vi "TEST_L1_TRANSFER_FUNCTION.vi"(5 "Serial Number":string="SN_00268", 6 "error in":errorcluster, 9 "Instrument VISA in":T1={"AWG VISA"="AgilentGen1", "Oscilloscope  VISA "="AgilentOsc", "Integration Board IP"="172.16.17.48", "connection ID"=refnum, "report out"=refnum, "report file path"=path "C:/Users/omartinez/Desktop/L0nL1_Results"}) -> (0 "error out":errorcluster, 3 "VISA Out":T1={"AWG VISA"="AgilentGen1", "Oscilloscope  VISA "="AgilentOsc", "Integration Board IP"="172.16.17.48", "connection ID"=refnum, "report out"=refnum, "report file path"=path "C:/Users/omartinez/Desktop/L0nL1_Results"})   [LabVIEW 2012]
uses:
  <vilib>/Utility/NIReport.llb/NI_report.lvclass
  <vilib>/Utility/NIReport.llb/HTML/NI_HTML.lvclass
  <instrlib>/Agilent 8000 Series/Agilent 8000 Series.lvlib
  Sum_Abrilader/L0_Sum_Adder Folder/C/Program Files/National Instruments/LabVIEW 2012/instr.lib/Agilent 81150/Agilent 81150.lvlib
panel:
  in  "SmartScan/\nLinearScan?":bool
  in  "Threshold Limits":i16[](array[numeric])=[0, 255]
  out "Threshold Limits":i32[](array[numeric])=[0, 1]
  in  "Gains":dbl[](array[numeric])=[0.96, 0.97, 0.98, 0.88, 1.0, 1.0, 0.99]
  out "Current Channel":i32
  in  "Pulse Amplitudes":dbl[](array[numeric])=[0.1, 0.4, 1.0]
  in  "Combination\n  (Act High)":i32 min=0 max=127 step=1 format="%b"
  in  "Single/Comb":bool=TRUE
  in  "Single Channel Enable":i32(slide) scale=0.0..6.0
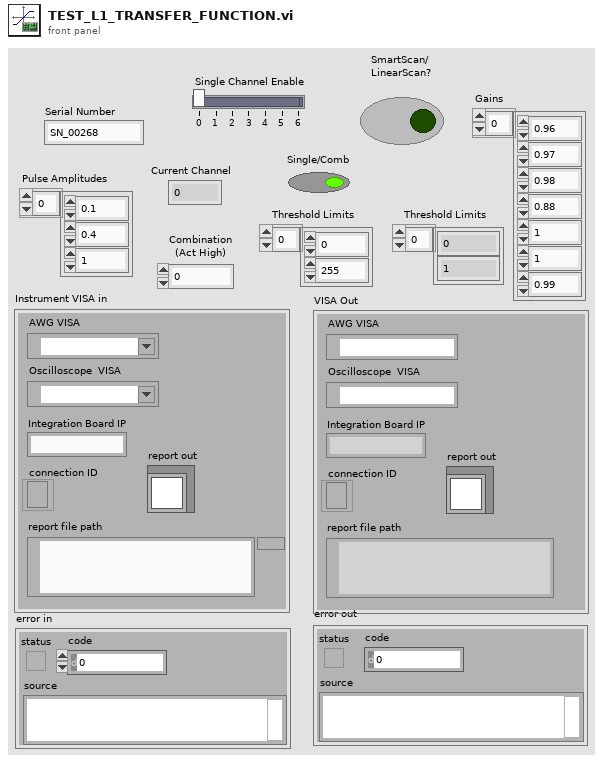
[diagram p1: front panel]
types:
  T1 = cluster{"AWG VISA":refnum<visa-resource-name>, "Oscilloscope  VISA ":refnum<visa-resource-name>, "Integration Board IP":string, "connection ID":refnum<k5>, "report out":refnum<class "NI_report.lvclass">, "report file path":path}
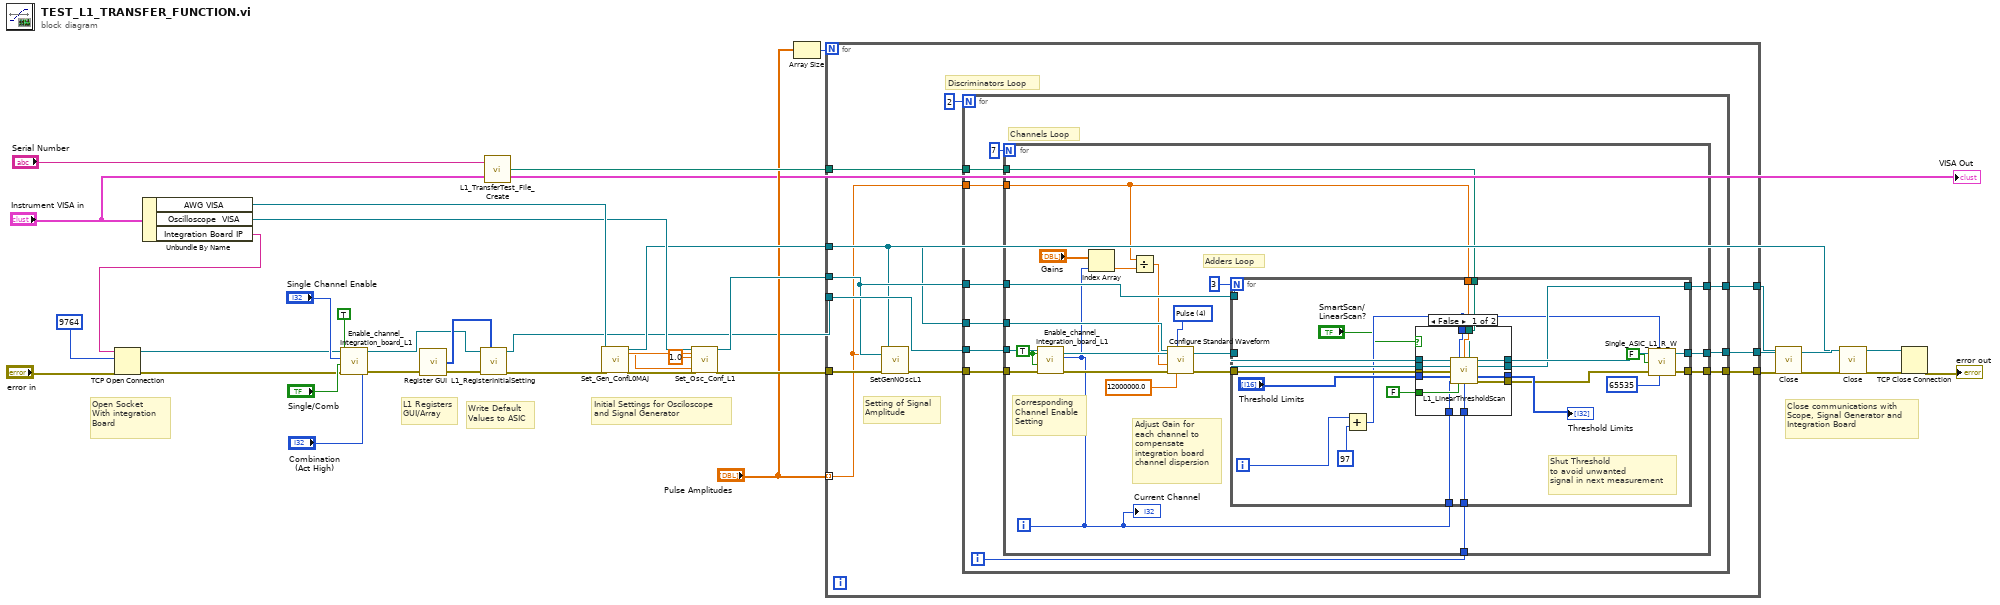
[diagram p0: block diagram]
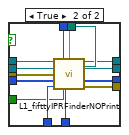
[diagram p2: hidden frame]
diagram:
  # "Write Default\nValues to ASIC"
  # "Close communications with \nScope, Signal Generator and \nIntegration Board"
  # "Initial Settings for Osciloscope\nand Signal Generator"
  # "L1 Registers\nGUI/Array"
  # "Open Socket\nWith integration \nBoard"
  n1 = Unbundle By Name("Instrument VISA in") -> ("AWG VISA"=w23:refnum<visa-resource-name>, "Oscilloscope  VISA"=w22:refnum<visa-resource-name>, "Integration Board IP"=w28:string)
  n2 = TCP Open Connection(address=w28, remote port or service name=9764, error in (no error)="error in") -> (connection ID=w10:refnum<k5>, error out=w1:errorcluster)  [unwired: 2 in]
  n3 = call "Enable_channel_Integration_board_L1.vi"("Combination"="Combination\n  (Act High)", "Enable  L1 single  Input"="Single Channel Enable", "error in (no error)"=w1, "SingleIN/#Combination"="Single/Comb", "Enable some/all"=TRUE ("#Enable all L1"), "connection ID"=w10) -> ("error out"=w2:errorcluster, "connection ID out"=w3:refnum<k5>)
  n4 = call "Register GUI.vi"("error in (no error)"=w2) -> ("error out"=w4:errorcluster, "REG ARRAy"=w5:u32[])  [unwired: 3 in]
  n5 = call "L1_RegisterInitialSetting.vi"("REG ARRAy"=w5, "error in"=w4, "connection ID in"=w3) -> ("error out"=w7:errorcluster, "connection ID out"=w6:refnum<k5>)  [unwired: 7 in]
  n6 = call "L1_TransferTest_File_Create.vi"("input cluster"="Instrument VISA in", "Serial Number"="Serial Number") -> ("appended path"=w27:path)
  n7 = call "Set_Gen_ConfL0MAJ.vi"("AWG VISA"=w23, "error in (no error)"=w7) -> ("Amplitude 1 OUT"=w25:dbl, "VISA resource name out"=w14:refnum<visa-resource-name>, "Pulse Width in seconds 1 OUT"=w24:dbl, "error out"=w26:errorcluster)  [unwired: 10 in, 4 out]
  n8 = call "Set_Osc_Conf_L1.vi"("VISA resource name"=w22, "Amplitude IN"=w25, "Trigger Level IN"=1.0, "Pulse Width in seconds IN"=w24, "error in (no error)"=w26) -> ("VISA resource name out"=w16:refnum<visa-resource-name>, "error out"=w17:errorcluster)  [unwired: 13 in]
  n9 = Array Size(array="Pulse Amplitudes") -> (size(s)=w13:i32)
  n10 = for {
    N: w13 -> [_]
    tunnel: [w46] -> w29
    tunnel: w27 -> [w45]
    tunnel: w6 -> [w44]
    tunnel: [w43] -> w21
    tunnel: [w42] -> w18
    tunnel: w17 -> [w41]
    tunnel: w16 -> [w39]
    tunnel: w14 -> [w38]
    tunnel: "Pulse Amplitudes" -> [w37] mode=indexing
    # "Discriminators Loop"
    # "Setting of Signal\nAmplitude"
    n11 = call "SetGenNOscL1.vi"("Input Voltage"=w37, "error in (no error)"=w41, "VISA resource name"=w39, "AWG VISA"=w38) -> ("error out 2"=w40:errorcluster)  [unwired: 7 in]
    n12 = for {
      N: 2 -> [_]
      tunnel: [w57] -> w46
      tunnel: w45 -> [w55]
      tunnel: w44 -> [w54]
      tunnel: [w53] -> w43
      tunnel: [w52] -> w42
      tunnel: w40 -> [w51]
      tunnel: w39 -> [w50]
      tunnel: w38 -> [w49]
      tunnel: w37 -> [w48]
      i -> [w47]
      # "Channels Loop"
      n13 = for {
        N: 7 -> [_]
        tunnel: [w78] -> w53
        tunnel: [w76] -> w57
        tunnel: w54 -> [w74]
        tunnel: w55 -> [w72]
        tunnel: w48 -> [w64]
        tunnel: w51 -> [w71]
        tunnel: w50 -> [w70]
        tunnel: [w69] -> w52
        tunnel: w49 -> [w65]
        tunnel: w47 -> [w58]
        i -> [w59]
        w68 = u16 4 items=["Sine", "Square", "Ramp Up", "Ramp Down", "Pulse", "Noise", "DC"] ("Waveform (0: Sine)")
        w73 = TRUE ("#Enable all L1")
        # "Adjust Gain for\neach channel to\ncompensate \nintegration board\nchannel dispersion"
        # "Corresponding\nChannel Enable\nSetting"
        # "Adders Loop"
        n14 = call "Enable_channel_Integration_board_L1.vi"("Enable  L1 single  Input"=w59, "error in (no error)"=w71, "SingleIN/#Combination"=w73, "Enable some/all"=w73, "connection ID"=w74) -> ("error out"=w67:errorcluster, "connection ID out"=w75:refnum<k5>)  [unwired: 1 in]
        n15 = Index Array(array="Gains", index=w59) -> (element=w60:dbl)
        n16 = Divide(x=w64, y=w60) -> (x/y=w63:dbl)
        n17 = call <instrlib>:"Configure Standard Waveform.vi"("Frequency (1000.0 Hz)"=12000000.0, "Waveform (0: Sine)"=w68, "error in (no error)"=w67, "Amplitude (1.0 Vpp)"=w63, "VISA resource name"=w65) -> ("error out"=w66:errorcluster)  [unwired: 5 in, 1 out]
        n18 = for {
          N: 3 -> [_]
          tunnel: w75 -> [w89]
          tunnel: w66 -> [w90]
          tunnel: [w97] -> w78
          tunnel: [w96] -> w76
          tunnel: w72 -> [w92]
          tunnel: w59 -> [w87]
          tunnel: w64 -> [w93]
          tunnel: w70 -> [w91]
          tunnel: [w83] -> w69
          tunnel: w58 -> [w82]
          i -> [w98]
          # "Shut Threshold\nto avoid unwanted\nsignal in next measurement"
          n19 = Add(x=w98, y=97) -> (x+y=w81:i32)
          n20 = case shown="False" "SmartScan/\nLinearScan?" {
            tunnel: w93 -> [w112 w127]
            tunnel: w92 -> [w110 w126]
            tunnel: w91 -> [w109 w125]
            tunnel: w90 -> [w107 w124]
            tunnel: w89 -> [w108 w123]
            tunnel: "Threshold Limits" -> [w106 w122]
            tunnel: w87 -> [w103 w121]
            tunnel: [w101 w120] -> w86
            tunnel: [w102 w119] -> w85
            tunnel: [w113 w118] -> w84
            tunnel: [w100 w117] -> w83
            tunnel: w82 -> [w104 w116]
            tunnel: w81 -> [w111 w115]
            tunnel: FALSE ("Adder Test?") -> [w105 w114]
            frame False {
              n21 = call "L1_LinearThresholdScan.vi"("VISA In"=w109, "Adder Register"=w111, "Vin"=w112, "File path In"=w110, "ID In"=w108, "Error In"=w107, "Threshold Limits In"=w106, "Channel/Mode"=w103, "Adder Test?"=w105, "Digital Output"=w104) -> ("ID out"=w113:refnum<k5>, "VISA Out"=w100:refnum<visa-resource-name>, "Threshold Limits Out"=w101:i16[], "Error Out"=w102:errorcluster)  [unwired: 2 in]
            }
            frame True {
              n22 = call "L1_fifttyIPRFinderNOPrint.vi"("VISA In"=w125, "Adder Register"=w115, "Vin"=w127, "File path In"=w126, "ID In"=w123, "Error In"=w124, "Threshold Limits In"=w122, "Channel/Mode"=w121, "Adder Test?"=w114, "Digital Output"=w116) -> ("ID out"=w118:refnum<k5>, "VISA Out"=w117:refnum<visa-resource-name>, "Threshold Limits Out"=w120:i16[], "Error Out"=w119:errorcluster)  [unwired: 2 in]
            }
          }
          "Threshold Limits" <- w86
          n23 = call "Single_ASIC_L1_R_W.vi"("connection ID"=w84, "Register or channel"=w81, "RD/#WR"=FALSE, "error in (no error)"=w85, "Data"=u32 65535 ("COMB DEC")) -> ("connection ID out"=w96:refnum<k5>, "error out"=w97:errorcluster)  [unwired: 1 in, 2 out]
        }
        "Current Channel" <- w59
      }
    }
  }
  n24 = call <instrlib>:"Close.vi"("error in (no error)"=w21, "VISA resource name"=w18) -> ("error out"=w20:errorcluster)  [unwired: 9 in]
  n25 = call <instrlib>:"Close.vi"("error in (no error)"=w20, "VISA resource name"=w14) -> ("error out"=w19:errorcluster)  [unwired: 9 in]
  n26 = TCP Close Connection(connection ID=w29, error in (no error)=w19) -> (error out=→"error out":errorcluster)  [unwired: 1 in, 1 out]
  "VISA Out" <- "Instrument VISA in"
